vi "Get Desired Size.vi"(8 "error in (no error)":errorcluster, 11 "DA Parent in":refnum<class "DA Parent.lvclass">) -> (0 "error out":errorcluster, 2 "Desired Size":T1, 3 "DA Parent out":refnum<class "DA Parent.lvclass">)   [LabVIEW 2020, in "Display As.lvlib" / "DA Parent.lvclass"]
uses:
  DA Parent.lvclass
  OOPanel/ArrayPanel/Desired Size.ctl
  OOPanel/ArrayPanel/ArrayPanel.lvclass
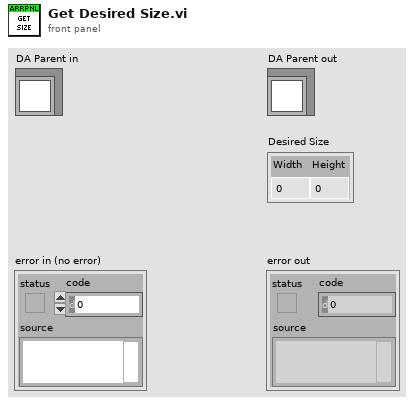
[diagram p1: front panel]
types:
  T1 = typedef "OOPanel.lvlib/ArrayPanel.lvclass/Desired Size.ctl" = cluster{"Width":u32, "Height":u32}
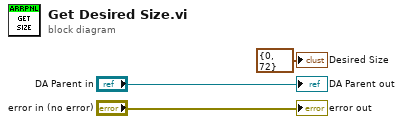
[diagram p0: block diagram]
diagram:
  "error out" <- "error in (no error)"
  "DA Parent out" <- "DA Parent in"
  "Desired Size" <- T1 {"Width"=0, "Height"=72} ("Desired Size")
